vi "Init_Test.vi"(8 "error in (no error)":errorcluster caption="entrée d'erreur (pas d'erreur)", 11 "Check_Func en entrée":refnum<class "Check_Func.lvclass">) -> (0 "error out":errorcluster caption="sortie d'erreur", 3 "Check_Func en sortie":refnum<class "Check_Func.lvclass">)   [LabVIEW 2020, in "Library Test.lvlib" / "Check_Func.lvclass"]
uses:
  Check_Func.lvclass
  C:/Users/ngarcin/OneDrive - Altyor/Standard TB/Class/Test/Test (Default)/Test (Default).lvclass
  Commun VI/TypeDef/Commande Test/Commande Type Test.ctl
  Commun VI/TypeDef/Commande Test/Commande Value Type.ctl
  Test_Without_Instr/Test_Without_Inst.lvclass
  Check_Func.lvclass/Check_Func.ctl
  Commun VI/Library Commun.lvlib
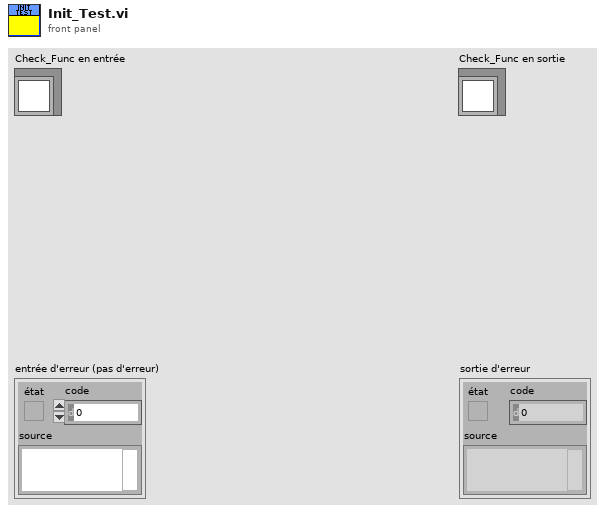
[diagram p1: front panel]
types:
  T1 = typedef "Library Commun.lvlib/Commande Value Type.ctl" = enum16{"None", "String", "Number", "Timestamp", "Boolean", "Array"}
  T2 = typedef "Library Commun.lvlib/Commande Type Test.ctl" = enum16{"Function", "Test", "Calculation"}
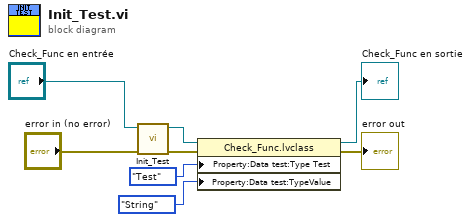
[diagram p0: block diagram]
diagram:
  n1 = call-parent "Init_Test.vi"("error in (no error)"="error in (no error)", "Test_Without_Inst en entrée"="Check_Func en entrée") -> ("error out"=w3:errorcluster, "Test_Without_Inst en sortie"=w5:refnum<class "Check_Func.lvclass">)  [unwired: 8 in]
  n2 = property class="Check_Func.lvclass"(reference=w5, error in=w3, "Property:Data test:Type Test"=Commande_Type_Test."Test" ("Type Test"), "Property:Data test:TypeValue"=Commande_Value_Type."String" ("TypeValue")) -> (reference out=→"Check_Func en sortie":refnum<class "Check_Func.lvclass">, error out=→"error out":errorcluster)
